vi "_Get Sheet.vi"(8 "error in":errorcluster, 10 "SheetName":string, 11 "SpreadsheetDocument in":refnum<k24>) -> (0 "error out":errorcluster, 3 "SpreadsheetDocument out":refnum<k24>)   [LabVIEW 2021, in "Open Xml.lvlib"]
uses:
  Open Xml.lvlib
  D:/git/Open-Xml-LabVIEW/dll/DocumentFormat.OpenXml.dll
  dll/DocumentFormat.OpenXml.dll
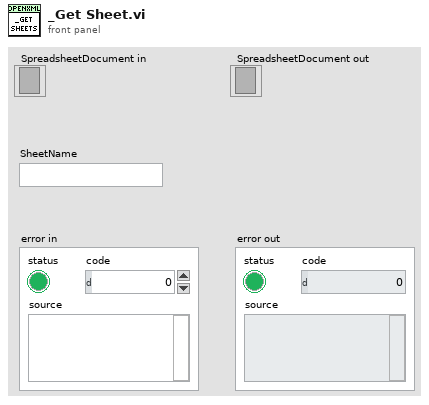
[diagram p1: front panel]
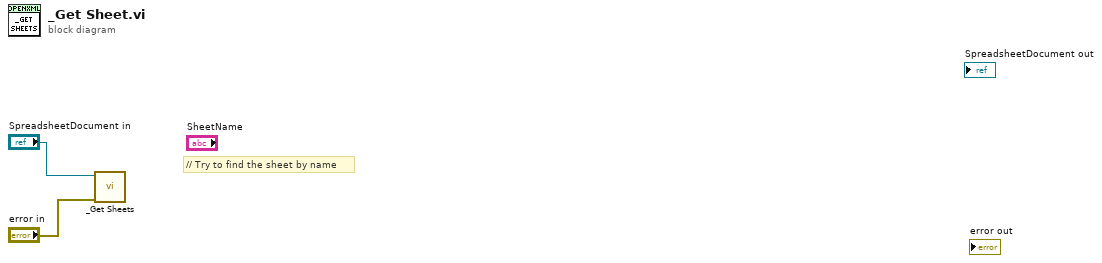
[diagram p0: block diagram]
diagram:
  # "// Try to find the sheet by name"
  n1 = call "_Get Sheets.vi"("error in"="error in", "SpreadsheetDocument in"="SpreadsheetDocument in") -> ()  [unwired: 8 in, 2 out]
